vi "GFGnumericGet.vi"(7 "GFG Refnum (use when calling from external project)":refnum<vi>, 8 "error in (no error)":errorcluster, 11 "Variable Name in":string) -> (0 "error out":errorcluster, 2 "Found/Replaced":bool, 3 "Numeric":dbl)   [LabVIEW 2012, in "GFG library.lvlib"]
doc: "SciScan 1.2 160622"
uses:
  GFG library.lvlib
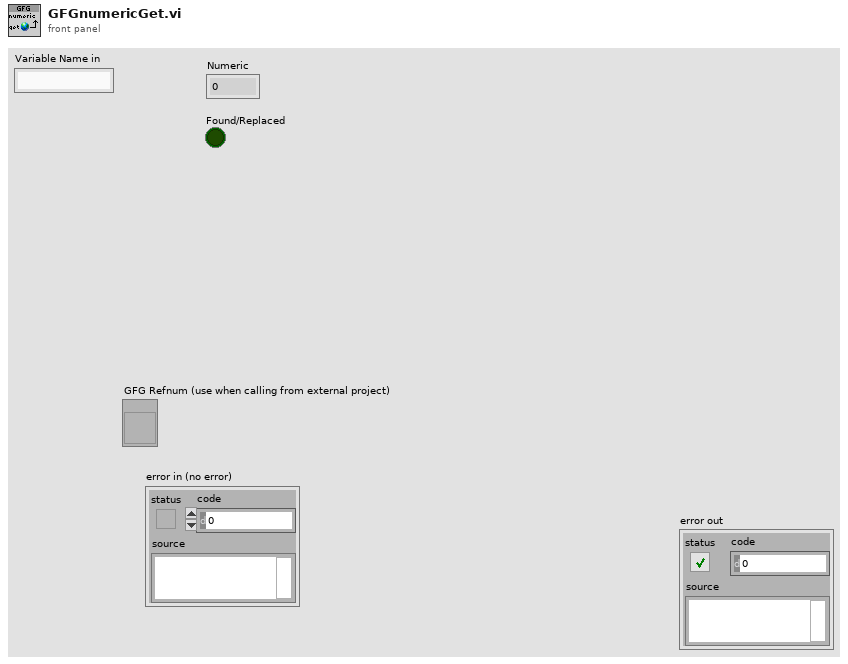
[diagram p1: front panel]
types:
  T1 = typedef "VariantType.lvlib/Type.ctl" = enum8{"Invalid Type", "Void", "I8", "I16", "I32", "I64", "U8", "U16", "U32", "U64", "Single Float", "Double Float", "Extended Float", "Single Complex", "Double Complex", "Extended Complex", "Enum U8", "Enum U16", "Enum U32", "Enum U64", "Single Float With Unit", "Double Float With Unit", "Extended Float With Unit", "Single Complex with Unit", "Double Complex with Unit", "Extended Complex with Unit", "Boolean", "String", "Path", "Picture", "Tag", "Array", "Cluster", "Variant", "LV Variant", "Waveform", "Timestamp", "Digital Waveform", "Digital Data", "ExpressData", "Refnum", "External Data", "VI", "Poly VI", "LabVIEW Class Instance", "Fixed Point"}
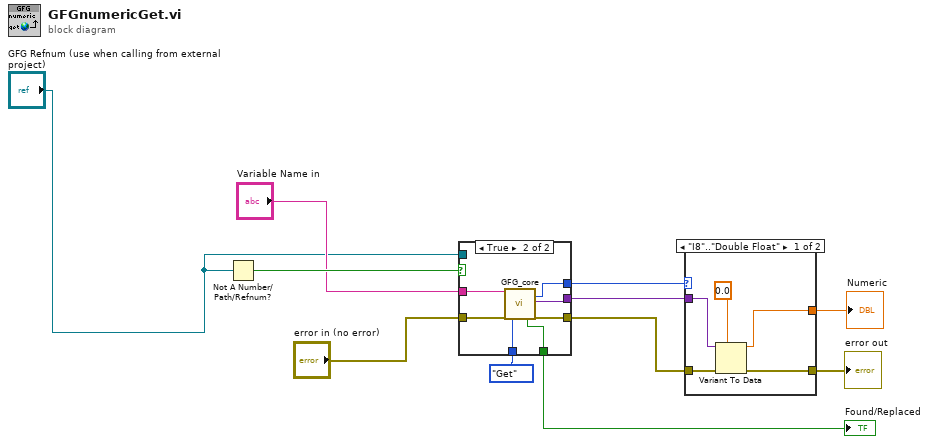
[diagram p0: block diagram]
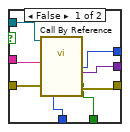
[diagram p2: hidden frame]
diagram:
  n1 = Not A Number/Path/Refnum?(number/path/refnum="GFG Refnum (use when calling from external project)") -> (NaN/Path/Refnum?=w8:bool)
  n2 = case shown="True" w8 {
    tunnel: enum16{"Init", "Set", "Get"}."Get" ("Action") -> [w14 w26]
    tunnel: "Variable Name in" -> [w15 w25]
    tunnel: "error in (no error)" -> [w19 w24]
    tunnel: [w18 w23] -> w5
    tunnel: [w16 w22] -> w3
    tunnel: [w17 w21] -> w4
    tunnel: "GFG Refnum (use when calling from external project)" -> [w13 _]
    tunnel: [w12 w20] -> w1
    frame False {
      n3 = call-by-ref "?"(reference=w13, "Variable Name in"=w15, "error in (no error)"=w19, "Action"=w14) -> ("Found/Replaced"=w12:bool, "Data Type Out"=w16:T1, "Variant Out"=w17:variant, "error out"=w18:errorcluster)  [unwired: 11 in, 5 out]
    }
    frame True {
      n4 = call "GFG_core.vi"("Variable Name in"=w25, "error in (no error)"=w24, "Action"=w26) -> ("Found/Replaced"=w20:bool, "Data Type Out"=w22:T1, "Variant Out"=w21:variant, "error out"=w23:errorcluster)  [unwired: 10 in, 3 out]
    }
  }
  "Found/Replaced" <- w1
  n5 = case shown="\"I8\"..\"Double Float\"" w3 {
    tunnel: w4 -> [w30 _]
    tunnel: [w29 _] -> w11
    tunnel: [w27 w32] -> w10
    tunnel: w5 -> [w28 w32]
    frame "I8".."Double Float" {
      n6 = Variant To Data(error in=w28, type=0.0, Variant=w30) -> (data=w29:dbl, error out=w27:errorcluster)
    }
    frame Default {
    }
  }
  "Numeric" <- w11
  "error out" <- w10
